vi "Read Accelerometer SPI.vi"(5 "gyro range (deg/sec)":u16(ring)=250 items=["250"=250, "500"=500, "1000"=1000, "2000"=2000], 6 "retries":u16=5, 7 "accel range (g)":u16(ring)=2 items=["2"=2, "4"=4, "8"=8, "16"=16], 8 "error in (no error)":errorcluster, 9 "check ready":bool=TRUE, 11 "Accelerometer":T2) -> (0 "error out":errorcluster, 2 "Accelerometer Data":T1, 3 "Accelerometer out":T2, 4 "num tries":i32)   [LabVIEW 2012]
doc: "Use this template to build a VI to use as a subVI."
uses:
  AccelerometerSPI.ctl
  <vilib>/ni845x/ni845x.llb/ni845xControl.ctl
  <vilib>/ni845x/ni845x.llb/ni845xSpiConfiguration.ctl
  Accelerometer Data.ctl
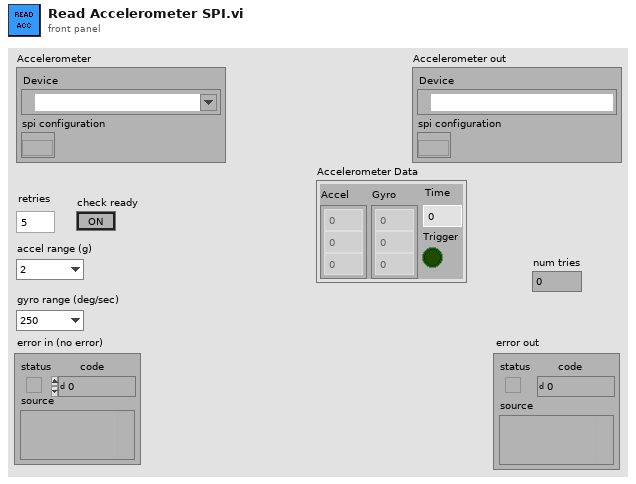
[diagram p1: front panel]
types:
  T1 = typedef "Accelerometer Data.ctl" = cluster{"Accel":dbl[], "Gyro":dbl[], "Time":u64, "Trigger":bool}
  T2 = typedef "AccelerometerSPI.ctl" = cluster{"Device":T3, "spi configuration":T4}
  T3 = typedef "ni845xControl.ctl" = refnum<k21>
  T4 = typedef "ni845xSpiConfiguration.ctl" = refnum<k20>
  T5 = typedef "ni845xDioLineWriteValue.ctl" = i32
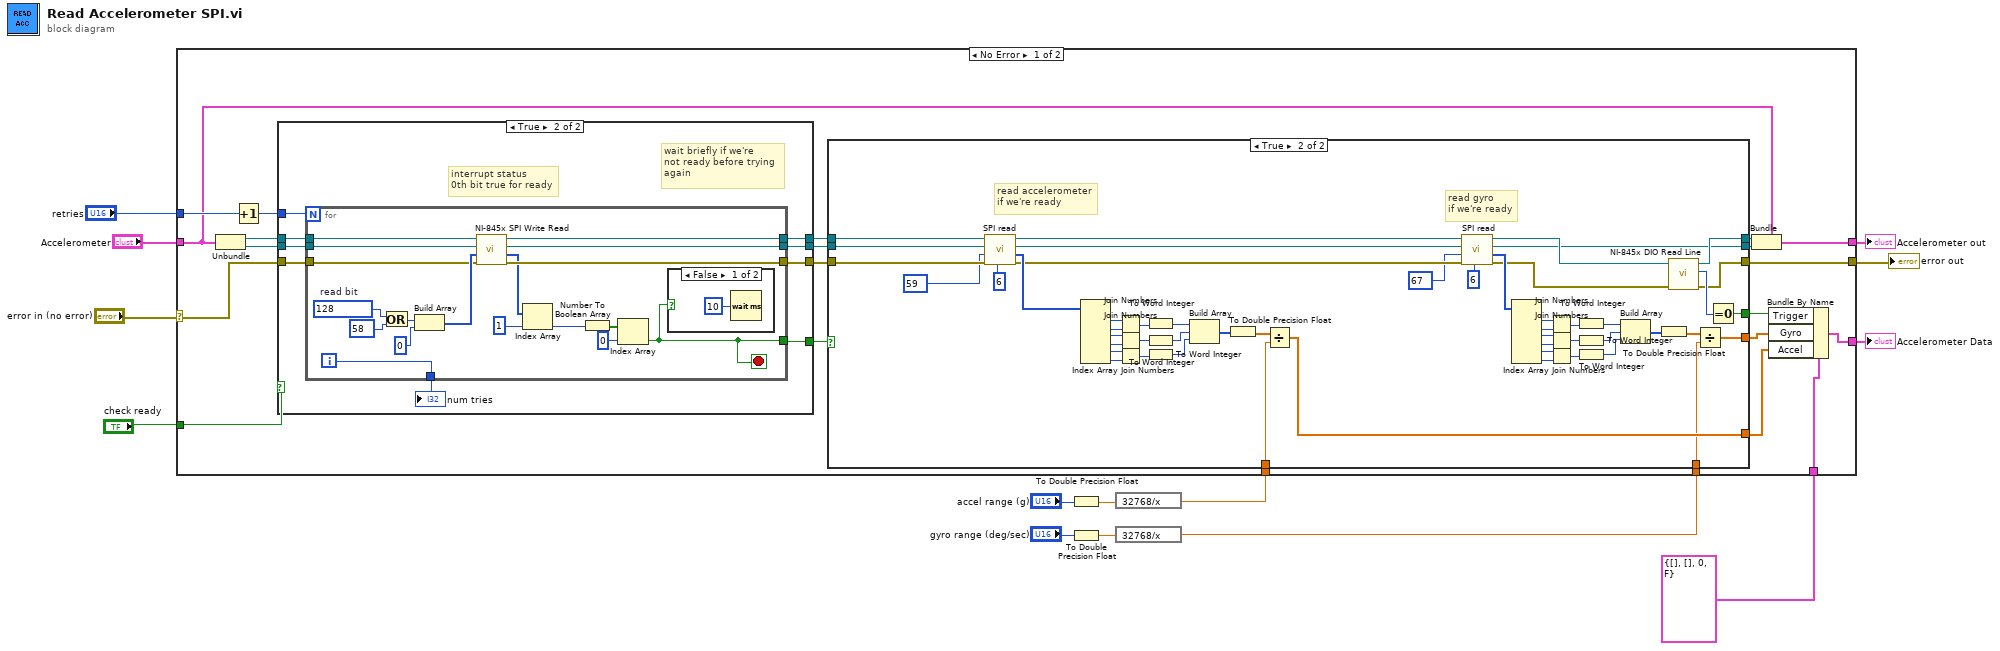
[diagram p0: block diagram]
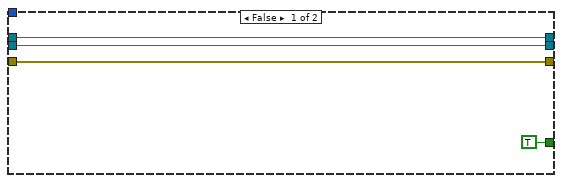
[diagram p2: hidden frame]
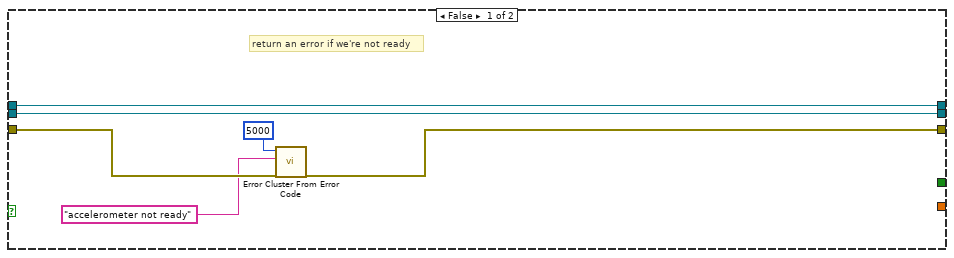
[diagram p4: hidden frame]
diagram:
  n1 = To Double Precision Float(number="accel range (g)") -> (double precision float=w7:dbl)
  n2 = To Double Precision Float(number="gyro range (deg/sec)") -> (double precision float=w6:dbl)
  n3 = expression code="32768/x"(w7) -> (w10:dbl)
  n4 = expression code="32768/x"(w6) -> (w5:dbl)
  n5 = case shown="No Error" "error in (no error)" {
    selector: "error in (no error)" -> [w32 w127]
    tunnel: [w35 w127] -> w13
    tunnel: "Accelerometer" -> [w22 w126]
    tunnel: [w23 w126] -> w11
    tunnel: w10 -> [w36 _]
    tunnel: "retries" -> [w30 _]
    tunnel: w5 -> [w21 _]
    tunnel: T1 {"Accel"=[], "Gyro"=[], "Time"=0, "Trigger"=FALSE} ("Accelerometer Data") -> [w20 _]
    tunnel: [w17 _] -> w2
    tunnel: "check ready" -> [w15 _]
    frame No Error {
      n6 = Unbundle(w22) -> ("Device"=w34:T3, "spi configuration"=w33:T4)
      n7 = Increment(x=w30) -> (x+1=w31:u16)
      n8 = case shown="True" w15 {
        tunnel: w34 -> [w40 w49]
        tunnel: w33 -> [w39 w48]
        tunnel: w32 -> [w38 w47]
        tunnel: w31 -> [_ w46]
        tunnel: [TRUE w45] -> w29
        tunnel: [w38 w44] -> w28
        tunnel: [w40 w43] -> w27
        tunnel: [w39 w42] -> w26
        frame False {
        }
        frame True {
          # "wait briefly if we're\nnot ready before trying\nagain"
          # "interrupt status\n0th bit true for ready"
          n9 = for {
            N: w46 -> [_]
            tunnel: w49 -> [w59]
            tunnel: w48 -> [w58]
            tunnel: [w64] -> w45
            tunnel: [w52] -> w43
            tunnel: [w53] -> w42
            tunnel: [w55] -> w44
            tunnel: w47 -> [w56]
            tunnel: [w63] -> w41
            i -> [w63]
            stop <- w64 stop-if-true
            w62 = u8 128  # read bit
            n10 = Or(x=w62, y=u8 58) -> (x .or. y?=w60:u8)
            n11 = Build Array(w60, u8 0 ("element")) -> (w57:u8[])
            n12 = call <vilib>:"NI-845x SPI Write Read.vi"("error in (no error)"=w56, "write data"=w57, "spi configuration in"=w58, "device reference in"=w59) -> ("error out"=w55:errorcluster, "read data"=w54:u8[], "spi configuration out"=w53:T4, "device reference out"=w52:T3)  [unwired: 4 in]
            n13 = Index Array(array=w54, index=1) -> (element=w67:u8)
            n14 = Number To Boolean Array(number=w67) -> (Boolean array=w66:bool[])
            n15 = Index Array(array=w66, index=0) -> (element=w64:bool)
            n16 = case shown="False" w64 {
              frame False {
                n17 = Wait (ms)(milliseconds to wait=u32 10) -> ()  [unwired: 1 out]
              }
              frame True {
              }
            }
          }
          "num tries" <- w41
        }
      }
      n18 = case shown="True" w29 {
        tunnel: w36 -> [_ w115]
        tunnel: [_ w110] -> w18
        tunnel: [w71 w92] -> w35
        tunnel: w28 -> [w74 w87]
        tunnel: w27 -> [w70 w89]
        tunnel: w26 -> [w69 w88]
        tunnel: [w70 w91] -> w25
        tunnel: [w69 w77] -> w24
        tunnel: w21 -> [_ w95]
        tunnel: [_ w94] -> w19
        tunnel: [_ w90] -> w16
        frame False {
          # "return an error if we're not ready"
          n19 = call <vilib>:"Error Cluster From Error Code.vi"("error in (no error)"=w74, "error message (\"\")"="accelerometer not ready" ("error message (\"\")"), "error code (0)"=5000) -> ("error out"=w71:errorcluster)  [unwired: 6 in]
        }
        frame True {
          # "read gyro\nif we're ready"
          # "read accelerometer\nif we're ready"
          n20 = call "SPI read.vi"("Number of bytes"=6, "error in (no error)"=w87, "Address"=u8 59, "spi configuration in"=w88, "Device ref in"=w89) -> ("error out"=w81:errorcluster, "read data"=w86:u8[], "spi configuration out"=w82:T4, "Device ref out"=w83:T3)  [unwired: 3 in]
          n21 = Index Array(array=w86) -> (element #1=w124:u8, element #2=w125:u8, element #3=w121:u8, element #4=w123:u8, element #5=w120:u8, element #6=w122:u8)  [unwired: 6 in]
          n22 = Join Numbers(hi=w124, lo=w125) -> ((hi.lo)=w118:u16)
          n23 = Join Numbers(hi=w121, lo=w123) -> ((hi.lo)=w117:u16)
          n24 = Join Numbers(hi=w120, lo=w122) -> ((hi.lo)=w116:u16)
          n25 = To Word Integer(number=w118) -> (16bit integer=w114:i16)
          n26 = To Word Integer(number=w117) -> (16bit integer=w113:i16)
          n27 = To Word Integer(number=w116) -> (16bit integer=w112:i16)
          n28 = Build Array(w114, w113, w112) -> (w111:i16[])
          n29 = To Double Precision Float(number=w111) -> (double precision float=w119:dbl[])
          n30 = Divide(x=w119, y=w115) -> (x/y=w110:dbl[])
          n31 = call "SPI read.vi"("Number of bytes"=6, "error in (no error)"=w81, "Address"=u8 67, "spi configuration in"=w82, "Device ref in"=w83) -> ("error out"=w75:errorcluster, "read data"=w76:u8[], "spi configuration out"=w77:T4, "Device ref out"=w78:T3)  [unwired: 3 in]
          n32 = Index Array(array=w76) -> (element #1=w97:u8, element #2=w96:u8, element #3=w100:u8, element #4=w98:u8, element #5=w101:u8, element #6=w99:u8)  [unwired: 6 in]
          n33 = Join Numbers(hi=w97, lo=w96) -> ((hi.lo)=w103:u16)
          n34 = Join Numbers(hi=w100, lo=w98) -> ((hi.lo)=w104:u16)
          n35 = Join Numbers(hi=w101, lo=w99) -> ((hi.lo)=w105:u16)
          n36 = To Word Integer(number=w103) -> (16bit integer=w106:i16)
          n37 = To Word Integer(number=w104) -> (16bit integer=w107:i16)
          n38 = To Word Integer(number=w105) -> (16bit integer=w108:i16)
          n39 = Build Array(w106, w107, w108) -> (w109:i16[])
          n40 = To Double Precision Float(number=w109) -> (double precision float=w102:dbl[])
          n41 = call <vilib>:"NI-845x DIO Read Line.vi"("error in (no error)"=w75, "device reference in"=w78) -> ("error out"=w92:errorcluster, "read value"=w93:T5, "device reference out"=w91:T3)  [unwired: 7 in]
          n42 = Divide(x=w102, y=w95) -> (x/y=w94:dbl[])
          n43 = Equal To 0?(x=w93) -> (x = 0?=w90:bool)
        }
      }
      n44 = Bundle(cluster=w22, "Device"=w25, "spi configuration"=w24) -> (w23:T2)
      n45 = Bundle By Name(cluster=w20, "Trigger"=w16, "Gyro"=w19, "Accel"=w18) -> (w17:T1)
    }
    frame Error {
    }
  }
  "error out" <- w13
  "Accelerometer out" <- w11
  "Accelerometer Data" <- w2
